vi "Call Param Selection By Reference.vi"(7 "Param Size":enum16{"Scalar", "1d", "2d"}(ring), 8 "error in (no error)":errorcluster, 9 "NIVS.System Definition Root":refnum<k24>, 10 "NodePath":string) -> (0 "error out":errorcluster, 2 "Selected NodePath":string)   [LabVIEW 2011]
uses:
  NationalInstruments.VeriStand.SystemStorage
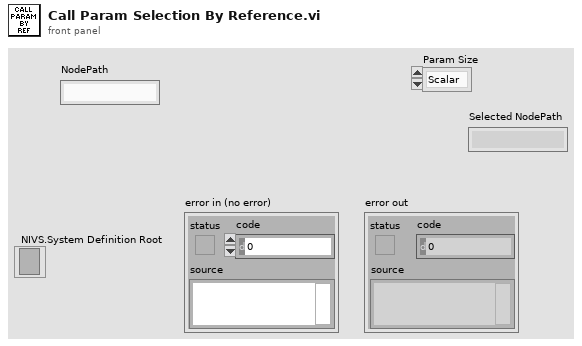
[diagram p1: front panel]
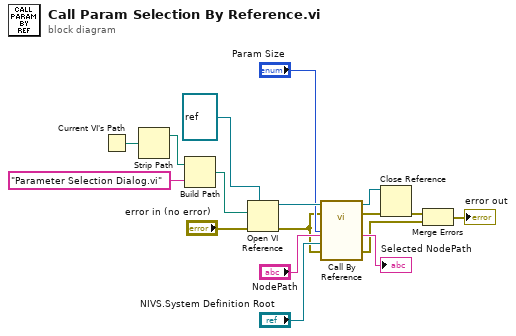
[diagram p0: block diagram]
diagram:
  n1 = Current VI's Path() -> (path=w17:path)
  n2 = Strip Path(path=w17) -> (stripped path=w2:path)  [unwired: 1 out]
  n3 = Build Path(base path=w2, name or relative path="Parameter Selection Dialog.vi") -> (appended path=w15:path)
  n4 = Open VI Reference(type specifier VI Refnum (for type only)=refnum<vi> refnum, vi path=w15, error in (no error)="error in (no error)") -> (vi reference=w13:refnum<vi>, error out=w9:errorcluster)  [unwired: 3 in]
  n5 = call-by-ref "?"(reference=w13, error in=w9, "Param Size"="Param Size", 8:"error in (no error)"=w9, "NIVS.System Definition Root"="NIVS.System Definition Root", "NodePath"="NodePath") -> (reference out=w5:refnum<vi>, error out=w4:errorcluster, 0:"error out"=w7:errorcluster, "Selected NodePath"=→"Selected NodePath":string)  [unwired: 6 in]
  n6 = Close Reference(reference=w5, error in (no error)=w4) -> (error out=w3:errorcluster)
  n7 = Merge Errors(w3, w7) -> (→"error out":errorcluster)
